vi "写入配置文件引用 i.vi"(8 "error in (no error)":errorcluster caption="错误输入（无错误）", 10 "配置文件引用":T1, 11 "段-输入":refnum<class "段-.lvclass">) -> (0 "error out":errorcluster caption="错误输出", 3 "段-输出":refnum<class "段-.lvclass">)   [LabVIEW 2017, in "项目开发助手.lvlib" / "模板-配置文件相关.lvlib" / "段-.lvclass"]
uses:
  <vilib>/Utility/config.llb/Config Data RefNum.ctl
  <vilib>/Utility/config.llb/NI_LVConfig.lvlib
panel:
  # "不需要重写此vi"
  # "配置文件由项目的配置文件模块打开, 然后将引用传入段实例\n所以不需要在此处打开文件, 否则多个配置文引用可能导致例不同步?"
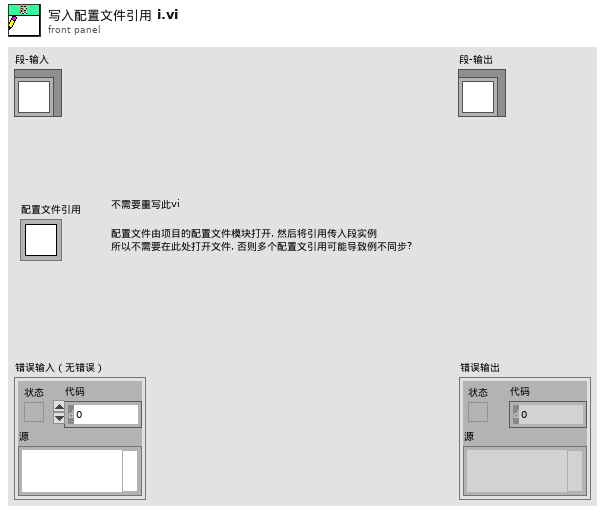
[diagram p1: front panel]
types:
  T1 = typedef "NI_LVConfig.lvlib/Config Data RefNum.ctl" = refnum<k1>
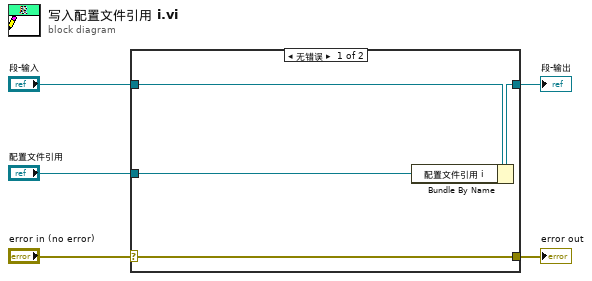
[diagram p0: block diagram]
diagram:
  n1 = case shown="无错误" "error in (no error)" {
    selector: "error in (no error)" -> [w9 w10]
    tunnel: [w9 w10] -> w4
    tunnel: [w7 w11] -> w2
    tunnel: "段-输入" -> [w8 w11]
    tunnel: "配置文件引用" -> [w6 _]
    frame No Error {
      n2 = Bundle By Name(cluster=w8, "配置文件引用 i"=w6) -> (w7:refnum<class "段-.lvclass">)
    }
    frame Error {
    }
  }
  "error out" <- w4
  "段-输出" <- w2
